vi "Process.vi"(8 "error in":errorcluster, 11 "Measurement.WavelengthSweeping.UI":refnum<class "Measurement.WavelengthSweeping.UI.lvclass">) -> (0 "error out":errorcluster, 3 "Measurement.WavelengthSweeping.UI out":refnum<class "Measurement.WavelengthSweeping.UI.lvclass">)   [LabVIEW 2017, in "Measurement.WavelengthSweeping.UI.lvclass"]
doc: "---------------------------------------------------------------\nJKI State Machine Objects™\nhttp://jki.net/state-machine-objects/\nCopyright (C) 2005-2015, JKI <info@jki.net>\nALL RIGHTS RESERVEDJKI State Machine Objects (SMO) 1.0.0.5\nJKI - JKI\nCopyright (c) 2016, JKI"
uses:
  Measurement.WavelengthSweeping.UI.lvclass
  D:/Program Files (x86)/National Instruments/LabVIEW 2017/vi.lib/JKI/JKI SMO/SMO/SMO.lvclass
  D:/Program Files (x86)/National Instruments/LabVIEW 2017/vi.lib/JKI/JKI SMO/SMO.UI/SMO.UI.lvclass
  <vilib>/JKI/JKI SMO/SMO/Typedefs/Parent Call--Enum.ctl
  Measurement.WavelengthSweeping/Typedefs/MeasuredData--Cluster.ctl
  Measurement.WavelengthSweeping/Measurement.WavelengthSweeping.lvclass
  D:/upwork/Laser Measurement Tool/Laser/project/Subsystems/Measurement/Measurement.lvclass
  Measurement.UI/Measurement.UI.lvclass
  <vilib>/JKI/JKI SMO/SMO/SMO.lvclass
  <vilib>/JKI/JKI SMO/SMO.UI/SMO.UI.lvclass
  Measurement/Measurement.lvclass
panel:
  in  "Clear Button":bool
  in  "Stop Button":bool
  in  "Pause Button":bool
  in  "Start Button":bool
  in  "Close Button":bool
  out "Initialized":bool
  out "Power monitor":cluster{"X":dbl, "Y":dbl}[](graph) caption="XY Graph - Light"
  out "SMU":cluster{"X":dbl, "Y":dbl}[](graph) caption="XY Graph - Light"
  out "LIA":cluster{"X":dbl, "Y":dbl}[](graph) caption="XY Graph - Light"
  # "For instructions on how to use the JKI State Machine Objects, examples and video tutorials, visit:\nhttp://jki.net/state-machine-objects/\n\nJKI State Machine Objects™\nhttp://jki.net/state-machine-objects/\nCopyright (C) 2005-2015, JKI <info@jki.net>\nALL RIGHTS RESERVED"
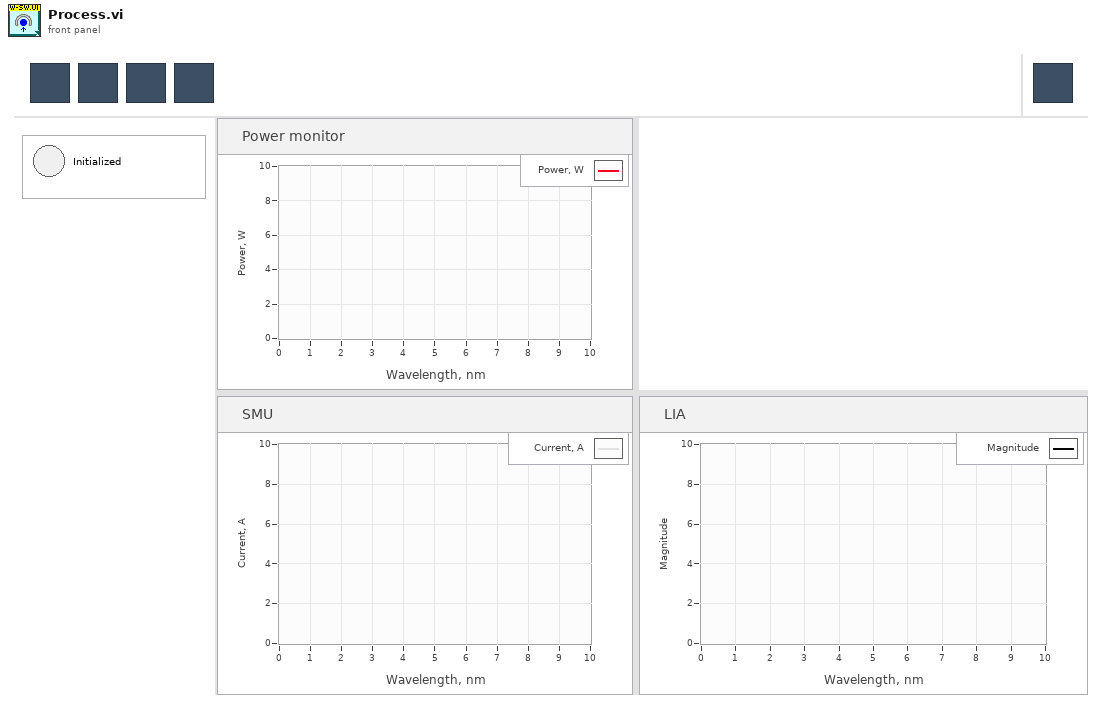
[diagram p1: front panel]
types:
  T1 = typedef "SMO.lvclass/Parent Call--Enum.ctl" = enum16{"Allows parent to run", "Does not request parent to run"}
  T2 = enum8{"Enabled", "Disabled", "Disabled and Grayed Out"}
  T3 = typedef "Measurement.WavelengthSweeping.lvclass/MeasuredData--Cluster.ctl" = cluster{"Wavelength, nm":dbl, "Power, W":dbl, "Current, A":dbl, "Magnitude":dbl}
  T4 = enum32{"invalid app kind", "Development System", "Run Time System", "Student Edition", "Embedded LabVIEW", "Evaluation", "Custom"}
  T5 = enum32{"Invalid", "Standard", "Closed", "Hidden", "Minimized", "Maximized"}
  T6 = typedef "Measurement.lvclass/PublicEvents--Measurement.Initialized.ctl" = bool
  T7 = typedef "Measurement.lvclass/PublicEvents--Measurement.Finished.ctl" = bool
  T8 = cluster{"Wavelength, nm":dbl, "Current, A":dbl}[]
  T9 = typedef "Measurement.WavelengthSweeping.UI.lvclass/Dependencies--Cluster.ctl" = cluster{"Measurement.WavelengthSweeping":refnum<class "Measurement.WavelengthSweeping.lvclass">}
  T10 = cluster{"Core":cluster{"Current VI Reference":refnum<vi>, "Close Panel on Exit?":bool, "error":errorcluster}, "Self Reference":refnum<class "Measurement.WavelengthSweeping.UI.lvclass">, "Dependencies":T9, "SMU Data":cluster{"X":dbl, "Y":dbl}[], "LIA Data":cluster{"X":dbl, "Y":dbl}[], "OPM Data":cluster{"X":dbl, "Y":dbl}[]}
  T11 = cluster{"Current VI Reference":refnum<vi>, "Close Panel on Exit?":bool, "error":errorcluster}
  T12 = typedef "SMO.lvclass/Protected Events.ctl" = cluster{"StopProcesses":refnum<user-event>, "AbortProcesses":refnum<user-event>, "Config Changed":refnum<user-event>, "Dependency":refnum<user-event>}
  T13 = cluster{"Event Registration Refnum":refnum<event-registration>, "Measurement Public Events":refnum<event-registration>}
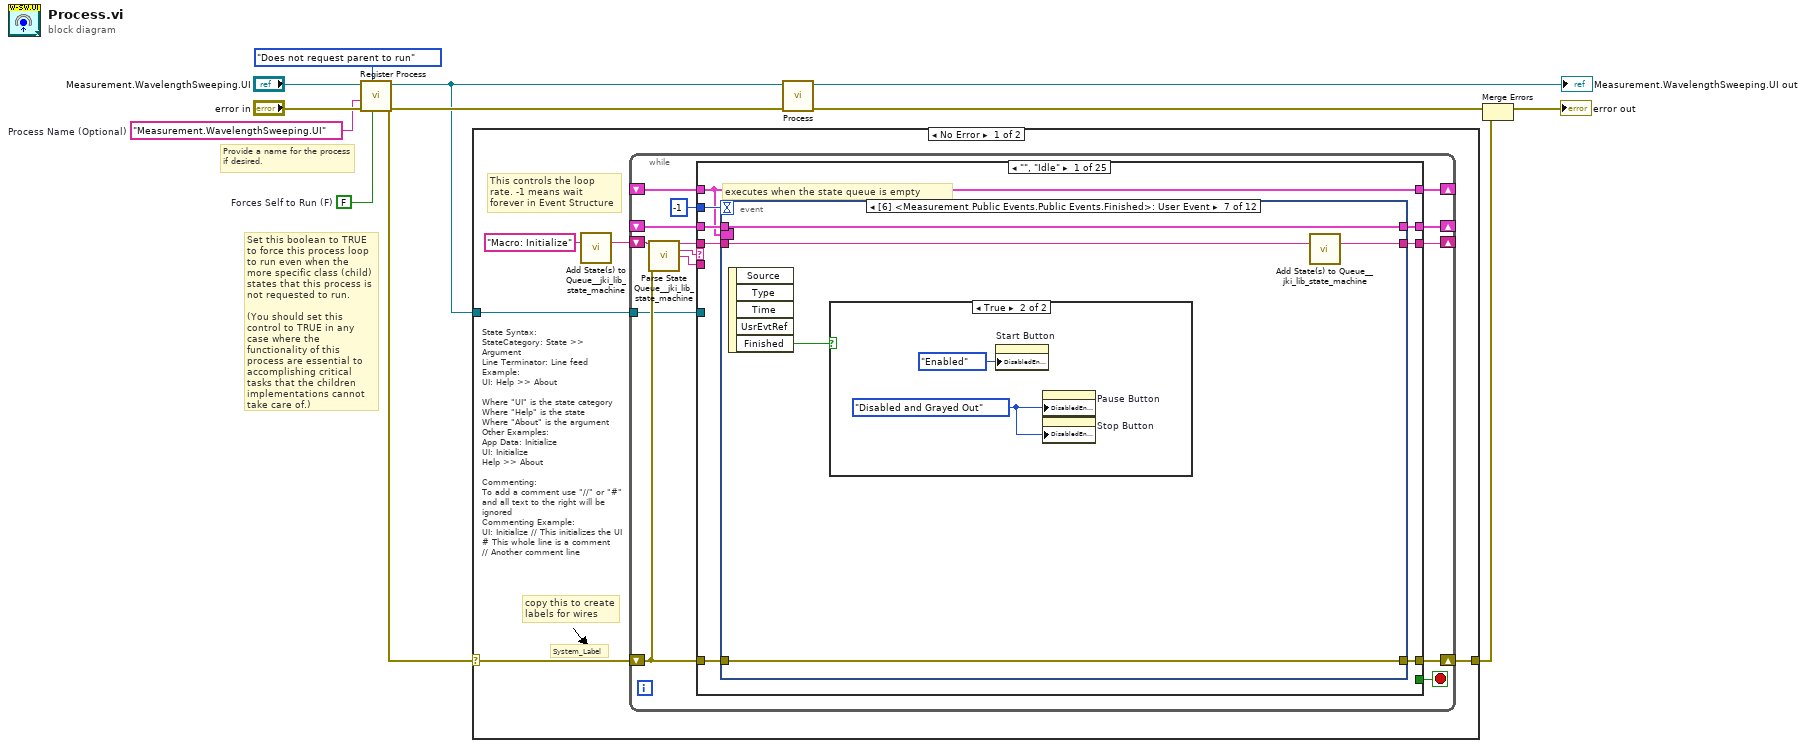
[diagram p0: block diagram]
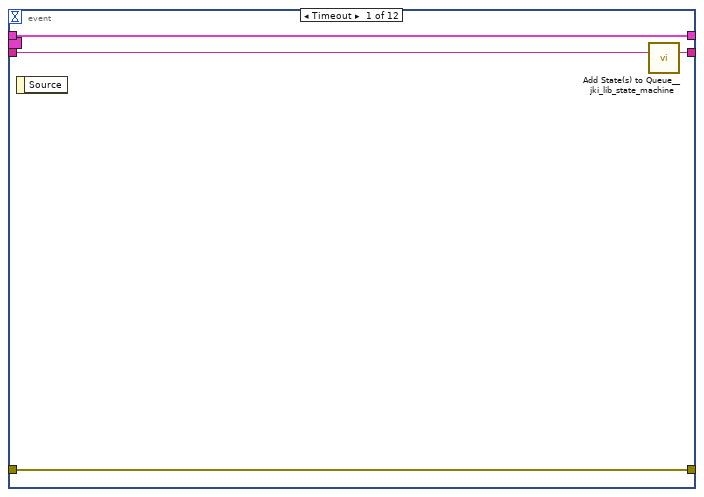
[diagram p2: hidden frame]
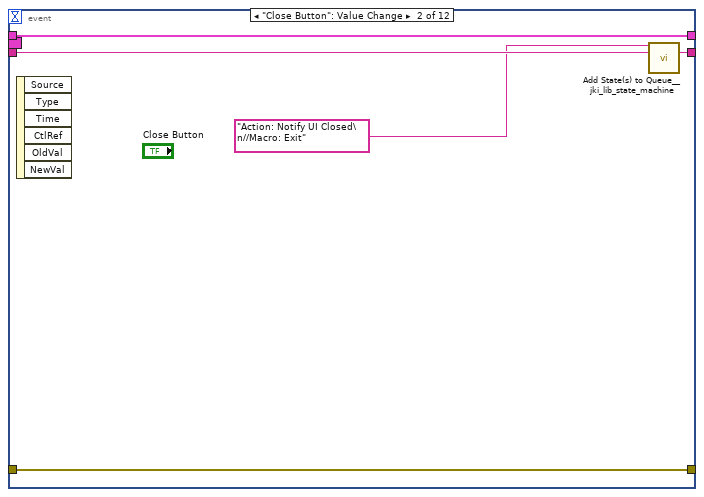
[diagram p3: hidden frame]
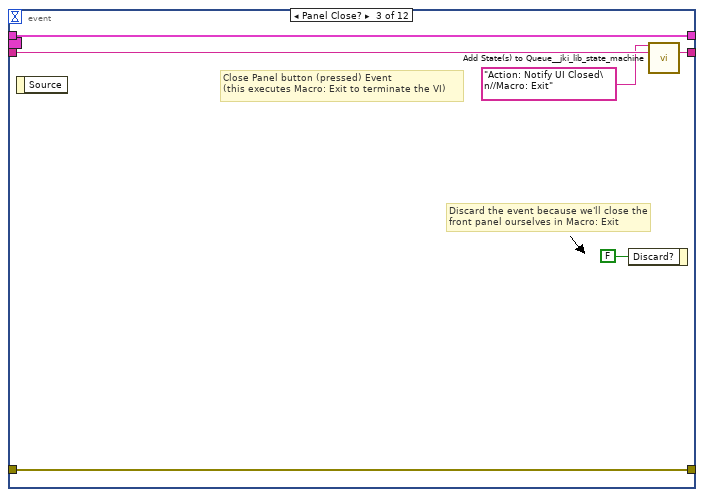
[diagram p4: hidden frame]
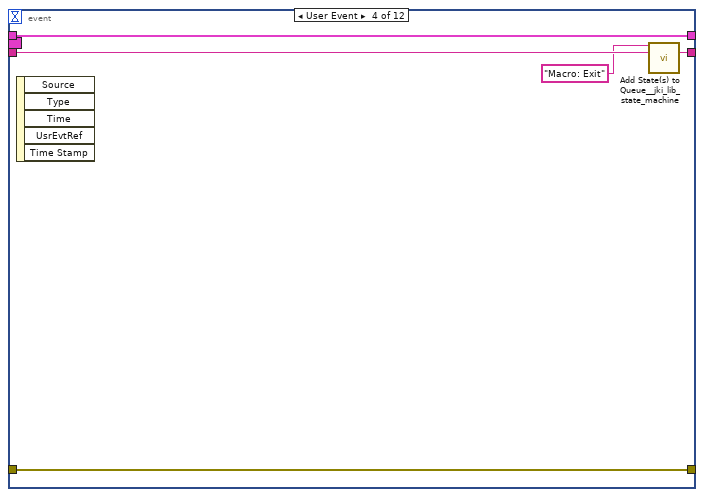
[diagram p5: hidden frame]
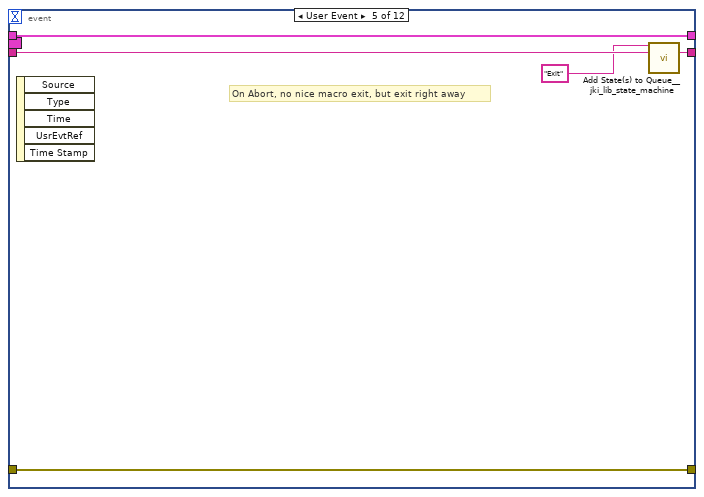
[diagram p6: hidden frame]
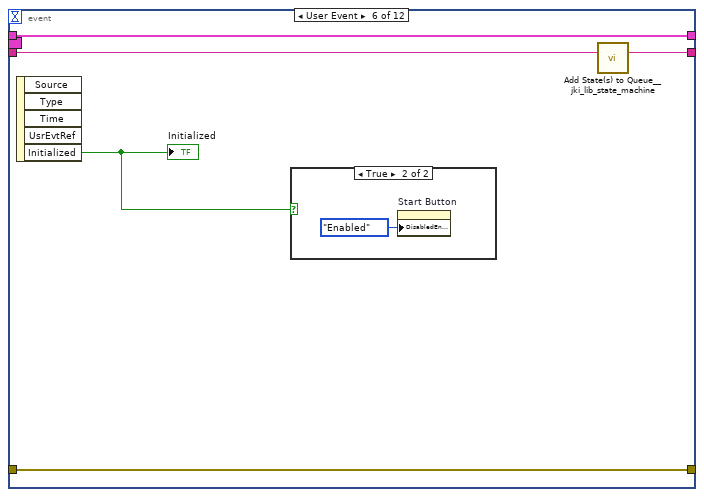
[diagram p7: hidden frame]
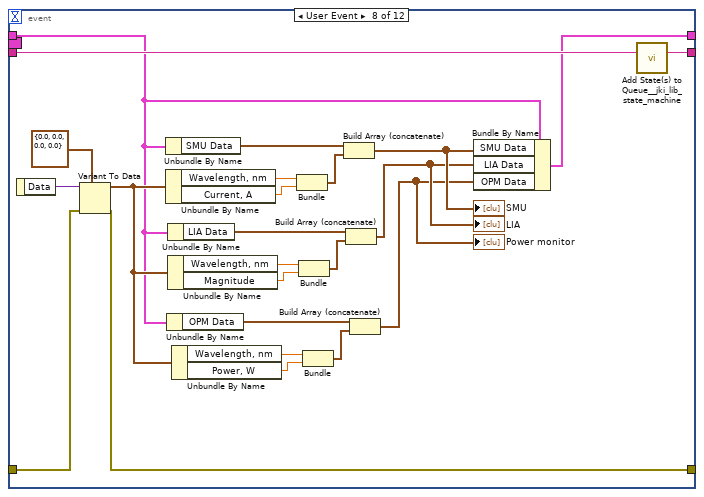
[diagram p10: hidden frame]
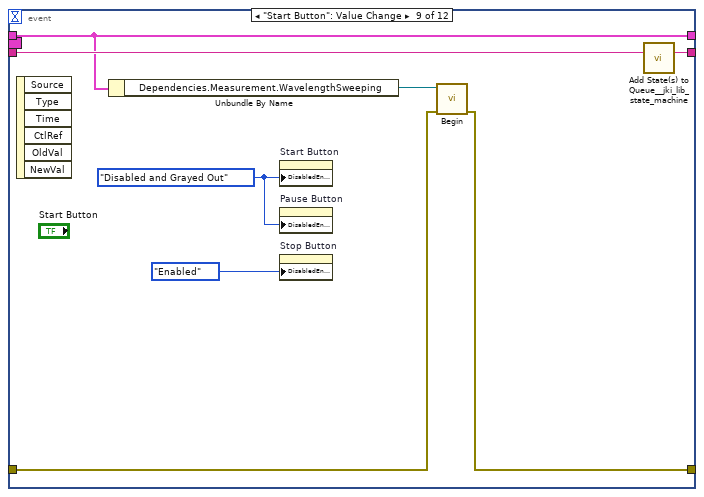
[diagram p11: hidden frame]
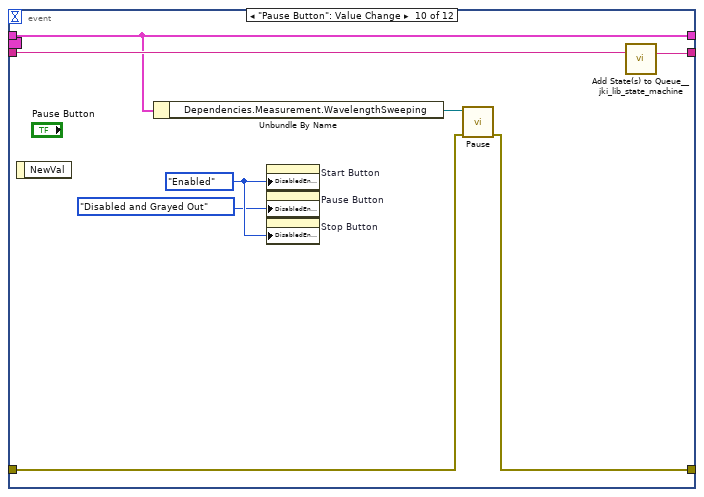
[diagram p12: hidden frame]
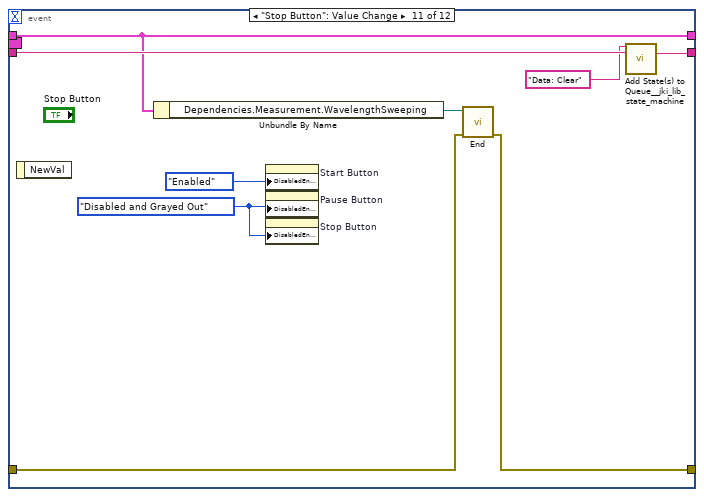
[diagram p13: hidden frame]
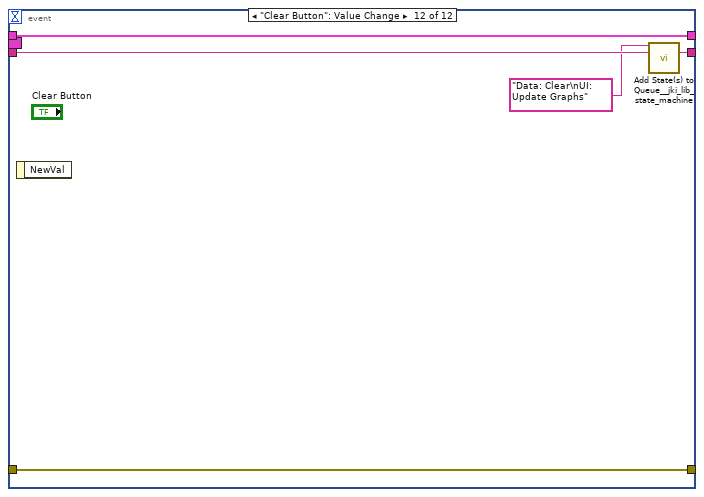
[diagram p14: hidden frame]
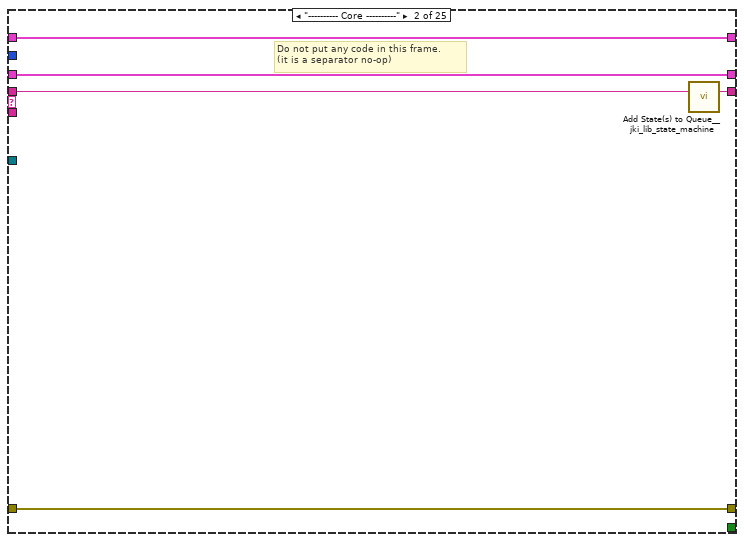
[diagram p15: hidden frame]
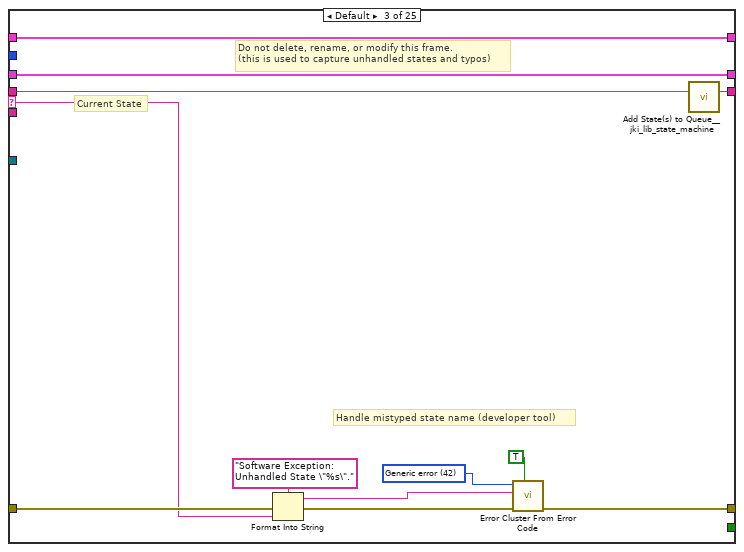
[diagram p16: hidden frame]
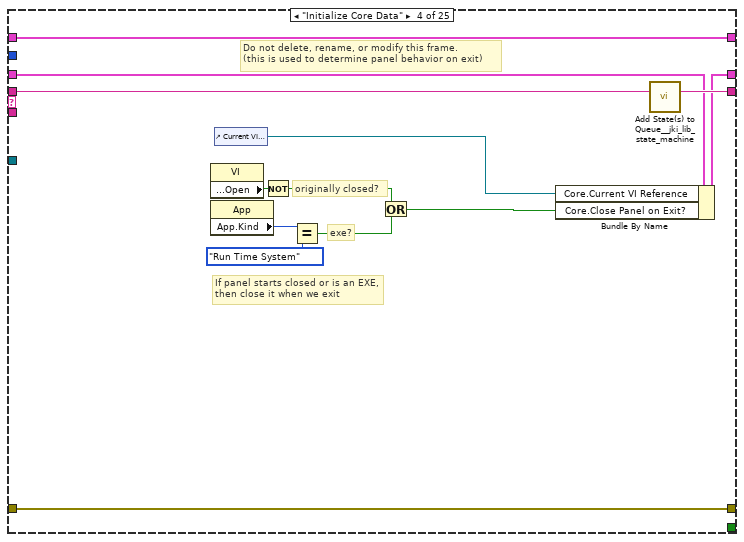
[diagram p17: hidden frame]
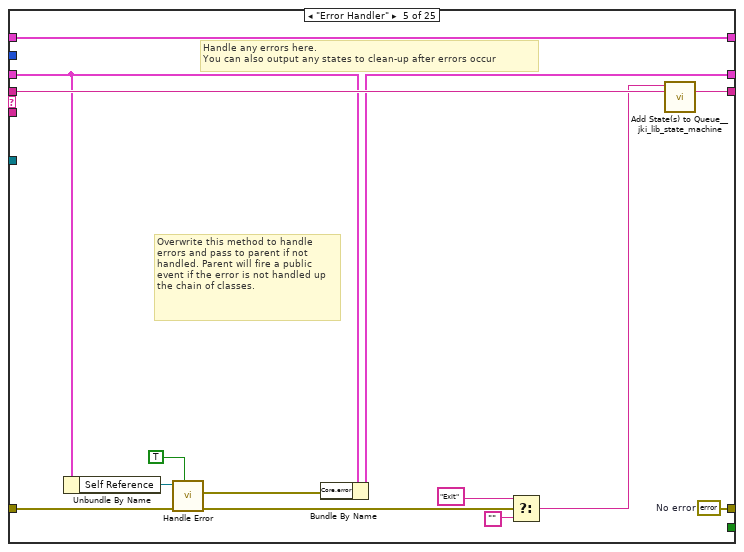
[diagram p18: hidden frame]
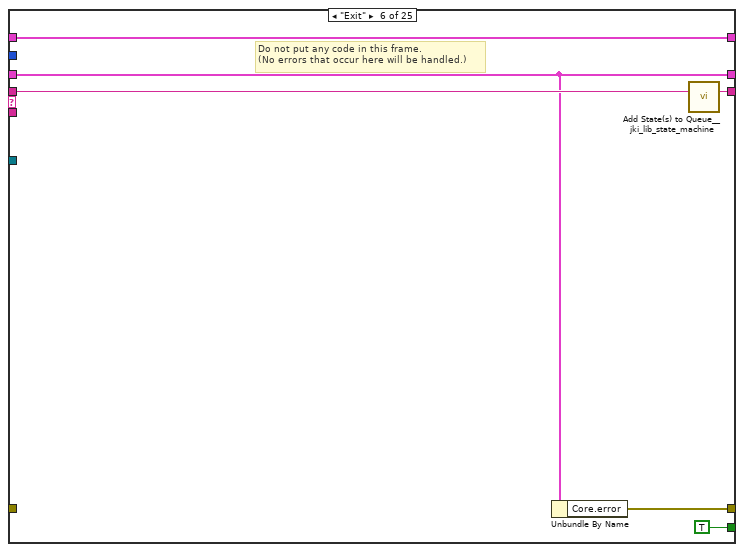
[diagram p19: hidden frame]
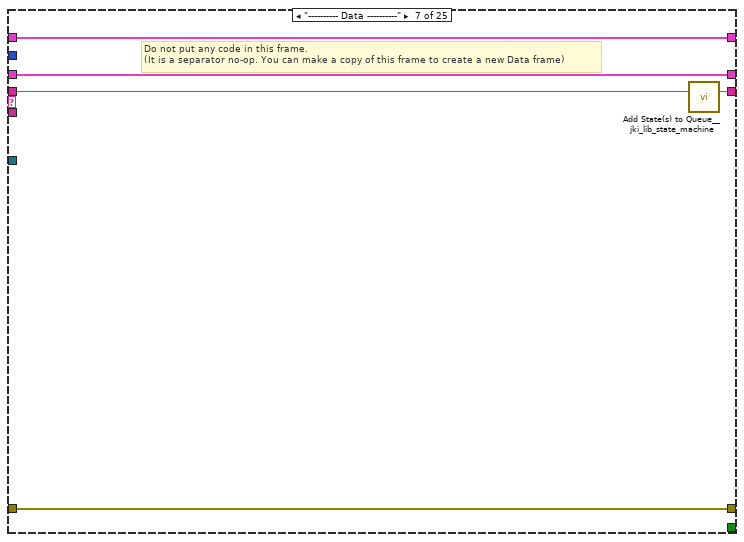
[diagram p20: hidden frame]
diagram:
  w2 = FALSE  # Forces Self to Run (F)
  w1 = "Measurement.WavelengthSweeping.UI"  # Process Name (Optional)
  # "Provide a name for the process\nif desired."
  # "Set this boolean to TRUE to force this process loop to run even when the more specific class (child) states that this process is not requested to run.\n\n(You should set this control to TRUE in any case where the functionality of this process are essential to accomplishing critical tasks that the children implementations cannot take care of.)"
  n1 = call <vilib>:"Register Process.vi"("Forces Self to Run (F)"=w2, "Parent Call"=Parent_Call--Enum."Does not request parent to run", "error in (no error)"="error in", "Process Name (optional)"=w1, "SMO"="Measurement.WavelengthSweeping.UI") -> ("error out"=w8:errorcluster, "SMO out"=w7:refnum<class "Measurement.WavelengthSweeping.UI.lvclass">)  [unwired: 5 in]
  n2 = case shown="No Error" w8 {
    selector: w8 -> [w13 w375]
    tunnel: w7 -> [w14 _]
    tunnel: [w12 w375] -> w4
    frame No Error {
      # "State Syntax:\nStateCategory: State >> Argument\nLine Terminator: Line feed\nExample:\nUI: Help >> About\n\nWhere \"UI\" is the state category\nWhere \"Help\" is the state\nWhere \"About\" is the argument\nOther Examples:\nApp Data: Initialize\nUI: Initialize\nHelp >> About\n\nCommenting:\nTo add a comment use \"//\" or \"#\" and all text to the right will be ignored\nCommenting Example:\nUI: Initialize // This initializes the UI\n# This whole line is a comment\n// Another comment line"
      # "copy this to create labels for wires"
      # "This controls the loop rate. -1 means wait forever in Event Structure"
      # "System_Label"
      n3 = call <vilib>:"Add State(s) to Queue__jki_lib_state_machine.vi"("State(s) in (\"\")"="Macro: Initialize") -> ("States Out"=w16:string)  [unwired: 14 in]
      n4 = while {
        shift-right: [w23] -> _
        shift-left: _ -> [w22]
        shift-right: [w26] -> w12
        shift-left: w13 -> [w20]
        shift-right: [w25] -> _
        shift-left: w16 -> [w27]
        tunnel: w14 -> [w19]
        shift-right: [w18] -> _
        shift-left: _ -> [w17]
        stop <- w24 stop-if-true
        n5 = call <vilib>:"Parse State Queue__jki_lib_state_machine.vi"("State Queue"=w27, "Error In (no error)"=w20) -> ("Remaining States"=w29:string, "Current State"=w30:string, "Arguments"=w28:string)  [unwired: 11 in]
        n6 = case shown="\"\", \"Idle\"" w30 {
          selector: w30 -> [_ _ w137 _ _ _ _ _ _ _ _ _ _ _ _ _ _ _ _ _ _ _ _ _ _]
          tunnel: w29 -> [w38 w135 w141 w160 w174 w180 w185 w200 w205 w214 w219 w229 w236 w252 w291 w296 w305 w319 w324 w335 w340 w354 w360 w367 w374]
          tunnel: w28 -> [_ _ _ _ _ _ _ _ _ _ _ _ w230 w246 _ _ _ _ _ _ _ _ _ _ _]
          tunnel: w22 -> [w36 w132 w139 w151 w163 w176 w182 _ w204 w209 w216 w227 w234 w248 w288 w293 w301 w310 w321 w332 w337 w346 w358 w363 w370]
          tunnel: [w35 w133 w143 w157 w165 w175 w183 w189 w202 w210 w217 w221 w231 w249 w280 w294 w303 w317 w322 w326 w338 w348 w355 w364 w368] -> w26
          tunnel: w20 -> [w34 w133 w142 w157 w170 _ w183 w197 w202 w211 w217 w225 w232 w250 w284 w294 w303 w317 w322 w327 w338 w350 w356 w364 w369]
          tunnel: [w37 w134 w140 w159 w173 w179 w184 w199 w206 w213 w218 w228 w235 w251 w290 w295 w304 w318 w323 w334 w339 w353 w359 w366 w373] -> w25
          tunnel: [_ _ _ _ _ TRUE _ _ _ _ _ _ _ _ _ _ _ _ _ _ _ _ _ _ _] -> w24
          tunnel: [w33 w132 w139 w158 w162 w176 w182 w198 w203 w209 w216 w227 w234 w248 w288 w293 w301 w310 w321 w332 w337 w346 w358 w362 w370] -> w23
          tunnel: -1 ("Timeout") -> [w32 _ _ _ _ _ _ _ _ _ _ _ _ _ _ _ _ _ _ _ _ _ _ _ _]
          tunnel: w19 -> [_ _ _ _ _ _ _ w195 _ _ _ _ _ _ _ _ _ _ _ _ _ _ _ _ _]
          tunnel: [w31 w131 w136 w148 w172 w177 w181 w194 w207 w208 w215 w226 w233 w245 w289 w292 w302 w311 w320 w333 w336 w343 w357 w365 w372] -> w18
          tunnel: w17 -> [w31 w131 w136 w148 w172 w177 w181 w194 w207 w208 w215 w226 w233 w245 w289 w292 w302 w311 w320 w333 w336 _ w357 w365 w372]
          frame "", "Idle" {
            # "executes when the state queue is empty"
            n7 = event shown="[6] <Measurement Public Events.Public Events.Finished>: User Event" {
              selector: w31 -> [_ _ _ _ _ _ _ _ _ _ _ _]
              dyn-events: _ -> [_ _ _ _ _ _ _ _ _ _ _ _]
              timeout: w32 -> [_ _ _ _ _ _ _ _ _ _ _ _]
              tunnel: w38 -> [w42 w47 w53 w58 w63 w65 w71 w99 w107 w115 w124 w130]
              tunnel: [w41 w46 w52 w57 w62 w66 w72 w100 w108 w116 w125 w129] -> w37
              tunnel: w36 -> [w39 w44 w49 w55 w60 w67 w73 w81 w106 w114 w123 w127]
              tunnel: [w40 w45 w48 w56 w61 w68 w74 w96 w103 w111 w120 w128] -> w35
              tunnel: w34 -> [w40 w45 w48 w56 w61 w68 w74 w97 w104 w112 w121 w128]
              tunnel: [w39 w44 w49 w55 w60 w67 w73 w80 w106 w114 w123 w127] -> w33
              event Timeout {
                n8 = event-data() -> ()  [unwired: 1 in, 1 out]
                n9 = call <vilib>:"Add State(s) to Queue__jki_lib_state_machine.vi"("State(s) in (\"\")"=w42) -> ("States Out"=w41:string)  [unwired: 14 in]
              }
              event "Close Button": Value Change {
                n10 = event-data() -> ()  [unwired: 1 in, 6 out]
                n11 = call <vilib>:"Add State(s) to Queue__jki_lib_state_machine.vi"("State(s) in Front (\"\")"="Action: Notify UI Closed\n//Macro: Exit" ("State(s) in Front (\"\")"), "State(s) in (\"\")"=w47) -> ("States Out"=w46:string)  [unwired: 13 in]
              }
              event Panel Close? {
                # "Discard the event because we'll close the front panel ourselves in Macro: Exit"
                # "Close Panel button (pressed) Event\n(this executes Macro: Exit to terminate the VI)"
                n12 = event-data() -> ()  [unwired: 1 in, 1 out]
                n13 = event-data("Discard?"=FALSE) -> ()  [unwired: 1 in, 1 out]
                n14 = call <vilib>:"Add State(s) to Queue__jki_lib_state_machine.vi"("State(s) in Front (\"\")"="Action: Notify UI Closed\n//Macro: Exit", "State(s) in (\"\")"=w53) -> ("States Out"=w52:string)  [unwired: 13 in]
              }
              event User Event {
                n15 = event-data() -> ()  [unwired: 1 in, 5 out]
                n16 = call <vilib>:"Add State(s) to Queue__jki_lib_state_machine.vi"("State(s) in Front (\"\")"="Macro: Exit", "State(s) in (\"\")"=w58) -> ("States Out"=w57:string)  [unwired: 13 in]
              }
              event User Event {
                # "On Abort, no nice macro exit, but exit right away"
                n17 = event-data() -> ()  [unwired: 1 in, 5 out]
                n18 = call <vilib>:"Add State(s) to Queue__jki_lib_state_machine.vi"("State(s) in Front (\"\")"="Exit", "State(s) in (\"\")"=w63) -> ("States Out"=w62:string)  [unwired: 13 in]
              }
              event User Event {
                n19 = event-data() -> ("Initialized"=w64:T6)  [unwired: 1 in, 4 out]
                "Initialized" <- w64
                n20 = case shown="True" w64 {
                  frame False {
                  }
                  frame True {
                    n21 = property on="Start Button" class="Bool"("DisabledEnum"=T2."Enabled" ("Disabled")) -> ()  [unwired: 2 in, 2 out]
                  }
                }
                n22 = call <vilib>:"Add State(s) to Queue__jki_lib_state_machine.vi"("State(s) in (\"\")"=w65) -> ("States Out"=w66:string)  [unwired: 14 in]
              }
              event User Event {
                n23 = event-data() -> ("Finished"=w70:T7)  [unwired: 1 in, 4 out]
                n24 = case shown="True" w70 {
                  frame False {
                  }
                  frame True {
                    w75 = T2."Disabled and Grayed Out" ("Disabled")
                    n25 = property on="Start Button" class="Bool"("DisabledEnum"=T2."Enabled" ("Disabled")) -> ()  [unwired: 2 in, 2 out]
                    n26 = property on="Pause Button" class="Bool"("DisabledEnum"=w75) -> ()  [unwired: 2 in, 2 out]
                    n27 = property on="Stop Button" class="Bool"("DisabledEnum"=w75) -> ()  [unwired: 2 in, 2 out]
                  }
                }
                n28 = call <vilib>:"Add State(s) to Queue__jki_lib_state_machine.vi"("State(s) in (\"\")"=w71) -> ("States Out"=w72:string)  [unwired: 14 in]
              }
              event User Event {
                n29 = event-data() -> ("Data"=w98:variant)  [unwired: 1 in]
                n30 = Variant To Data(error in=w97, type=T3 {"Wavelength, nm"=0.0, "Power, W"=0.0, "Current, A"=0.0, "Magnitude"=0.0} ("Measured Data"), Variant=w98) -> (data=w82:T3, error out=w96:errorcluster)
                n31 = Unbundle By Name(w81) -> ("SMU Data"=w92:cluster{"X":dbl, "Y":dbl}[])
                n32 = Unbundle By Name(w82) -> ("Wavelength, nm"=w94:dbl, "Current, A"=w93:dbl)
                n33 = Unbundle By Name(w81) -> ("OPM Data"=w84:cluster{"X":dbl, "Y":dbl}[])
                n34 = Unbundle By Name(w81) -> ("LIA Data"=w89:cluster{"X":dbl, "Y":dbl}[])
                n35 = Unbundle By Name(w82) -> ("Wavelength, nm"=w87:dbl, "Magnitude"=w88:dbl)
                n36 = Unbundle By Name(w82) -> ("Wavelength, nm"=w86:dbl, "Power, W"=w85:dbl)
                n37 = Bundle("Wavelength, nm"=w94, "Current, A"=w93) -> (w91:cluster{"Wavelength, nm":dbl, "Current, A":dbl})  [unwired: 1 in]
                n38 = Bundle("Wavelength, nm"=w87, "Magnitude"=w88) -> (w90:cluster{"Wavelength, nm":dbl, "Magnitude":dbl})  [unwired: 1 in]
                n39 = Bundle("Wavelength, nm"=w86, "Power, W"=w85) -> (w83:cluster{"Wavelength, nm":dbl, "Power, W":dbl})  [unwired: 1 in]
                n40 = Build Array (concatenate)(w92, w91) -> (w79:T8)
                "SMU" <- w79
                n41 = Build Array (concatenate)(w89, w90) -> (w78:cluster{"Wavelength, nm":dbl, "Magnitude":dbl}[])
                "LIA" <- w78
                n42 = Build Array (concatenate)(w84, w83) -> (w77:cluster{"Wavelength, nm":dbl, "Power, W":dbl}[])
                "Power monitor" <- w77
                n43 = Bundle By Name(cluster=w81, "SMU Data"=w79, "LIA Data"=w78, "OPM Data"=w77) -> (w80:T10)
                n44 = call <vilib>:"Add State(s) to Queue__jki_lib_state_machine.vi"("State(s) in (\"\")"=w99) -> ("States Out"=w100:string)  [unwired: 14 in]
              }
              event "Start Button": Value Change {
                w101 = T2."Disabled and Grayed Out" ("Disabled")
                n45 = event-data() -> ()  [unwired: 1 in, 6 out]
                n46 = Unbundle By Name(w106) -> ("Dependencies.Measurement.WavelengthSweeping"=w105:refnum<class "Measurement.WavelengthSweeping.lvclass">)
                n47 = property on="Start Button" class="Bool"("DisabledEnum"=w101) -> ()  [unwired: 2 in, 2 out]
                n48 = property on="Pause Button" class="Bool"("DisabledEnum"=w101) -> ()  [unwired: 2 in, 2 out]
                n49 = property on="Stop Button" class="Bool"("DisabledEnum"=T2."Enabled" ("Disabled")) -> ()  [unwired: 2 in, 2 out]
                n50 = call "Begin.vi"("error in (no error)"=w104, "Measurement in"=w105) -> ("error out"=w103:errorcluster)  [unwired: 8 in, 1 out]
                n51 = call <vilib>:"Add State(s) to Queue__jki_lib_state_machine.vi"("State(s) in (\"\")"=w107) -> ("States Out"=w108:string)  [unwired: 14 in]
              }
              event "Pause Button": Value Change {
                w110 = T2."Enabled" ("Disabled")
                n52 = event-data() -> ()  [unwired: 1 in, 1 out]
                n53 = Unbundle By Name(w114) -> ("Dependencies.Measurement.WavelengthSweeping"=w113:refnum<class "Measurement.WavelengthSweeping.lvclass">)
                n54 = property on="Start Button" class="Bool"("DisabledEnum"=w110) -> ()  [unwired: 2 in, 2 out]
                n55 = property on="Pause Button" class="Bool"("DisabledEnum"=T2."Disabled and Grayed Out" ("Disabled")) -> ()  [unwired: 2 in, 2 out]
                n56 = property on="Stop Button" class="Bool"("DisabledEnum"=w110) -> ()  [unwired: 2 in, 2 out]
                n57 = call "Pause.vi"("error in (no error)"=w112, "Measurement in"=w113) -> ("error out"=w111:errorcluster)  [unwired: 8 in, 1 out]
                n58 = call <vilib>:"Add State(s) to Queue__jki_lib_state_machine.vi"("State(s) in (\"\")"=w115) -> ("States Out"=w116:string)  [unwired: 14 in]
              }
              event "Stop Button": Value Change {
                w118 = T2."Disabled and Grayed Out" ("Disabled")
                n59 = event-data() -> ()  [unwired: 1 in, 1 out]
                n60 = Unbundle By Name(w123) -> ("Dependencies.Measurement.WavelengthSweeping"=w122:refnum<class "Measurement.WavelengthSweeping.lvclass">)
                n61 = property on="Start Button" class="Bool"("DisabledEnum"=T2."Enabled" ("Disabled")) -> ()  [unwired: 2 in, 2 out]
                n62 = property on="Pause Button" class="Bool"("DisabledEnum"=w118) -> ()  [unwired: 2 in, 2 out]
                n63 = property on="Stop Button" class="Bool"("DisabledEnum"=w118) -> ()  [unwired: 2 in, 2 out]
                n64 = call "End.vi"("error in (no error)"=w121, "Measurement in"=w122) -> ("error out"=w120:errorcluster)  [unwired: 8 in, 1 out]
                n65 = call <vilib>:"Add State(s) to Queue__jki_lib_state_machine.vi"("State(s) in Front (\"\")"="Data: Clear", "State(s) in (\"\")"=w124) -> ("States Out"=w125:string)  [unwired: 13 in]
              }
              event "Clear Button": Value Change {
                n66 = event-data() -> ()  [unwired: 1 in, 1 out]
                n67 = call <vilib>:"Add State(s) to Queue__jki_lib_state_machine.vi"("State(s) in Front (\"\")"="Data: Clear\nUI: Update Graphs", "State(s) in (\"\")"=w130) -> ("States Out"=w129:string)  [unwired: 13 in]
              }
            }
          }
          frame "---------- Core ----------" {
            # "Do not put any code in this frame.\n(it is a separator no-op)"
            n68 = call <vilib>:"Add State(s) to Queue__jki_lib_state_machine.vi"("State(s) in (\"\")"=w135) -> ("States Out"=w134:string)  [unwired: 14 in]
          }
          frame Default {
            w146 = 42 items=["No error", "Argument error", "Memory is full", "Out of zone", "End of file", "File already open", "Generic file I/O error", "File not found", "File permission error", "Disk is full", "Duplicate path", "Too many files open", "System feature not enabled", "Resource file not found", "Cannot add resource", "Resource not found", "Image not found", "Image memory error", "Pen does not exist", "Config type invalid", "Config token not found", "Config parse error", "Config memory error", "Bad external code format", "Bad external code offset", "External code not present", "Null window", "Destroy window error", "Null menu", "Print aborted", "Bad print record", "Print driver error", "Windows error during printing", "Memory error during printing", "Print dialog error", "Generic print error", "Invalid device refnum", "Device not found", "Device parameter error", "Device unit error", "Cannot open device", "Device call aborted", "Generic error", "Cancelled by user", "Object ID too low", "Object ID too high", "Object not in heap", "Unknown heap", "Unknown object (invalid DefProc)", "Unknown object (DefProc not in table)", "Message out of range", "Invalid (null) method", "Unknown message", "Manager call not supported", "Bad address", "Network operation in progress", "Network operation timed out", "Connection is busy", "Network attribute not supported", "Network error", "Address in use", "System out of memory", "Connection aborted", "Connection refused", "Not connected", "Already connected", "Connection closed", "Initialization error (interapplication manager)", "Bad occurrence", "Wait on unbound occurrence handler", "Occurrence queue overflow", "Datalog type conflict", "Unused", "Unrecognized type (interapplication manager)", "Memory corrupt", "Failed to make temporary DLL", "Old CIN version", "Drag socket not found", "Failed to load drop-object", "Failed to register OLE object", "Failed to release OLE object", "Format specifier type mismatch", "Unknown format specifier", "Too few format specifiers", "Too many format specifiers", "Scan failed", "Newer CIN version", "Error converting to variant", "Runtime menu error", "Password tampered", "Variant attribute not found", "Incompatible variant data type", "Event data is not available", "Event Store is not present", "Occurrence is not found", "Event Queue is not created", "Event info is not available", "Refnum passed is NULL", "Error retrieving Class GUID", "Error retrieving CoClass GUID", "Error retrieving TypeLib GUID.", "Bad built application magic bytes.", "Specific driver is different from the specific driver associated with the Logical Name.", "There is no session opened to the class driver.", "Max Error", "MAX - Error with config objects", "MAX - Error loading configuration", "MAX - Group not supported"]
            # "Current State"
            # "Do not delete, rename, or modify this frame.\n(this is used to capture unhandled states and typos)"
            # "Handle mistyped state name (developer tool)"
            n69 = Format Into String(format string="Software Exception: Unhandled State \"%s\"." ("message"), error in=w142, w137) -> (resulting string=w145:string, error out=w144:errorcluster)  [unwired: 1 in]
            n70 = call <vilib>:"Error Cluster From Error Code.vi"("show call chain? (False)"=TRUE, "error in (no error)"=w144, "error message (\"\")"=w145, "error code (0)"=w146) -> ("error out"=w143:errorcluster)  [unwired: 5 in]
            n71 = call <vilib>:"Add State(s) to Queue__jki_lib_state_machine.vi"("State(s) in (\"\")"=w141) -> ("States Out"=w140:string)  [unwired: 14 in]
          }
          frame "Initialize Core Data" {
            # "Do not delete, rename, or modify this frame.\n(this is used to determine panel behavior on exit)"
            # "originally closed?"
            # "exe?"
            # "If panel starts closed or is an EXE, then close it when we exit"
            n72 = property class="VI"() -> ("Front Panel.Open"=w156:bool)  [unwired: 2 in, 2 out]
            n73 = property class="App"() -> ("App.Kind"=w155:T4)  [unwired: 2 in, 2 out]
            n74 = control-ref of="Current VI Reference"() -> (w149:refnum<vi>)
            n75 = Not(x=w156) -> (.not. x?=w153:bool)
            n76 = Equal?(x=w155, y=T4."Run Time System" ("Application:Kind")) -> (x = y?=w152:bool)
            n77 = Or(x=w153, y=w152) -> (x .or. y?=w150:bool)
            n78 = Bundle By Name(cluster=w151, "Core.Current VI Reference"=w149, "Core.Close Panel on Exit?"=w150) -> (w158:T10)
            n79 = call <vilib>:"Add State(s) to Queue__jki_lib_state_machine.vi"("State(s) in (\"\")"=w160) -> ("States Out"=w159:string)  [unwired: 14 in]
          }
          frame "Error Handler" {
            w165 = errorcluster {"status"=FALSE, "code"=0, "source"=""}  # No error
            # "Overwrite this method to handle errors and pass to parent if not handled. Parent will fire a public event if the error is not handled up the chain of classes."
            # "Handle any errors here.\nYou can also output any states to clean-up after errors occur"
            n80 = Unbundle By Name(w163) -> ("Self Reference"=w171:refnum<class "Measurement.WavelengthSweeping.UI.lvclass">)
            n81 = call-dynamic "Handle Error.vi"("Stop on Unhandled Error (T)"=TRUE, "error in"=w170, "SMO"=w171) -> ("handling error"=w166:errorcluster, "Unhandled error"=w164:errorcluster)  [unwired: 6 in, 1 out]
            n82 = Bundle By Name(cluster=w163, "Core.error"=w164) -> (w162:T10)
            n83 = Select(t="Exit", s=w166, f="") -> (s? t:f=w167:string)
            n84 = call <vilib>:"Add State(s) to Queue__jki_lib_state_machine.vi"("State(s) in Front (\"\")"=w167, "State(s) in (\"\")"=w174) -> ("States Out"=w173:string)  [unwired: 13 in]
          }
          frame "Exit" {
            # "Do not put any code in this frame.\n(No errors that occur here will be handled.)"
            n85 = Unbundle By Name(w176) -> ("Core.error"=w175:errorcluster)
            n86 = call <vilib>:"Add State(s) to Queue__jki_lib_state_machine.vi"("State(s) in (\"\")"=w180) -> ("States Out"=w179:string)  [unwired: 14 in]
          }
          frame "---------- Data ----------" {
            # "Do not put any code in this frame.\n(It is a separator no-op. You can make a copy of this frame to create a new Data frame)"
            n87 = call <vilib>:"Add State(s) to Queue__jki_lib_state_machine.vi"("State(s) in (\"\")"=w185) -> ("States Out"=w184:string)  [unwired: 14 in]
          }
          frame "Data: Initialize" {
            w186 = cluster{"X":dbl, "Y":dbl}[] []  # OPM Data
            w187 = cluster{"X":dbl, "Y":dbl}[] []  # LIA Data
            w188 = cluster{"X":dbl, "Y":dbl}[] []  # SMU Data
            w193 = T11 {"Current VI Reference"=refnum, "Close Panel on Exit?"=FALSE, "error"={"status"=FALSE, "code"=0, "source"=""}}  # Core
            w196 = refnum<class "Measurement.WavelengthSweeping.UI.lvclass"> refnum  # Self Reference
            # "do not delete - used by framework"
            # "Data names and types of shift register data are defined by this bundle."
            # "Initialize the shift-register data, here.\n(data names are defined by what you wire into the bundle function)"
            n88 = Variant To Data(error in=w197, type=w196, Variant=w195) -> (data=w192:refnum<class "Measurement.WavelengthSweeping.UI.lvclass">, error out=w190:errorcluster)
            n89 = call "Measurement.WavelengthSweeping.UI.GetDependencies.vi"("error in (no error)"=w190, "Measurement.WavelengthSweeping.UI in"=w192) -> ("error out"=w189:errorcluster, "Dependencies"=w191:T9)  [unwired: 7 in, 1 out]
            n90 = Bundle("Core"=w193, "Self Reference"=w192, "Dependencies"=w191, "SMU Data"=w188, "LIA Data"=w187, "OPM Data"=w186) -> (w198:T10)  [unwired: 1 in]
            n91 = call <vilib>:"Add State(s) to Queue__jki_lib_state_machine.vi"("State(s) in (\"\")"=w200) -> ("States Out"=w199:string)  [unwired: 14 in]
          }
          frame "Data: Clear" {
            w201 = cluster{"X":dbl, "Y":dbl}[] [] ("SMU Data")
            n92 = Bundle By Name(cluster=w204, "SMU Data"=w201, "LIA Data"=w201, "OPM Data"=w201) -> (w203:T10)
            n93 = call <vilib>:"Add State(s) to Queue__jki_lib_state_machine.vi"("State(s) in (\"\")"=w205) -> ("States Out"=w206:string)  [unwired: 14 in]
          }
          frame "Data: Cleanup" {
            # "Cleanup any data and references, here.\n(this is called automatically, by the Macro: Exit)"
            n94 = Unbundle By Name(w209) -> ("Core.Current VI Reference"=w212:refnum<vi>)
            n95 = Close Reference(reference=w212, error in (no error)=w211) -> (error out=w210:errorcluster)
            n96 = call <vilib>:"Add State(s) to Queue__jki_lib_state_machine.vi"("State(s) in (\"\")"=w214) -> ("States Out"=w213:string)  [unwired: 14 in]
          }
          frame "---------- UI ----------" {
            # "Do not put any code in this frame.\n(It is a separator no-op. You can make a copy of this frame to create a new UI frame)"
            n97 = call <vilib>:"Add State(s) to Queue__jki_lib_state_machine.vi"("State(s) in (\"\")"=w219) -> ("States Out"=w218:string)  [unwired: 14 in]
          }
          frame "UI: Initialize" {
            w220 = T2."Disabled and Grayed Out" ("Disabled")
            # "Initialize the User Interface, here.\n(this is called automatically, by the Macro: Init)"
            n98 = invoke on="Initialized" class="Bool (strict)" method="Reinit To Default"(error in=w225) -> (error out=w222:errorcluster)  [unwired: 2 in, 2 out]
            n99 = invoke on="Power monitor" class="XYGraph (strict)" method="Reinit To Default"(error in=w222) -> (error out=w224:errorcluster)  [unwired: 2 in, 2 out]
            n100 = property on="Start Button" class="Bool"("DisabledEnum"=w220) -> ()  [unwired: 2 in, 2 out]
            n101 = property on="Pause Button" class="Bool"("DisabledEnum"=w220) -> ()  [unwired: 2 in, 2 out]
            n102 = property on="Stop Button" class="Bool"("DisabledEnum"=w220) -> ()  [unwired: 2 in, 2 out]
            n103 = invoke on="SMU" class="XYGraph (strict)" method="Reinit To Default"(error in=w224) -> (error out=w223:errorcluster)  [unwired: 2 in, 2 out]
            n104 = invoke on="LIA" class="XYGraph (strict)" method="Reinit To Default"(error in=w223) -> (error out=w221:errorcluster)  [unwired: 2 in, 2 out]
            n105 = call <vilib>:"Add State(s) to Queue__jki_lib_state_machine.vi"("State(s) in (\"\")"=w229) -> ("States Out"=w228:string)  [unwired: 14 in]
          }
          frame "UI: Cursor Set" {
            # "Argument"
            # "Initialize the User Interface, here.\n(this is called automatically, by the Macro: Init)"
            n106 = disable-structure shown="Default" {
              disable-tunnel: w232 -> [w237 w240]
              disable-tunnel: [w237 w239] -> w231
              disable-tunnel: w230 -> [_ w238]
              frame condition #0 {
              }
              frame condition #1 (active) {
                n107 = case shown="\"Idle\", Default" w238 {
                  tunnel: w240 -> [w242 w244]
                  tunnel: [w241 w243] -> w239
                  frame "Idle", Default {
                    n108 = call <vilib>:"Unset Busy.vi"("error in (no error)"=w242) -> ("error out"=w241:errorcluster)  [unwired: 10 in]
                  }
                  frame "Busy" {
                    n109 = call <vilib>:"Set Busy.vi"("error in (no error)"=w244) -> ("error out"=w243:errorcluster)  [unwired: 9 in, 1 out]
                  }
                }
              }
            }
            n110 = call <vilib>:"Add State(s) to Queue__jki_lib_state_machine.vi"("State(s) in (\"\")"=w236) -> ("States Out"=w235:string)  [unwired: 14 in]
          }
          frame "UI: Front Panel State" {
            # "Argument"
            # "Set Front Panel Open or Closed\n(Usage: \"UI: Front Panel State >> Open|Close\")"
            n111 = Unbundle By Name(w248) -> ("Core.Current VI Reference"=w247:refnum<vi>)
            n112 = disable-structure shown="Default" {
              disable-tunnel: w250 -> [w256 w279]
              disable-tunnel: [w255 w279] -> w249
              disable-tunnel: w247 -> [w254 _]
              disable-tunnel: w246 -> [w253 _]
              frame condition #0 (active) {
                n113 = case shown="\"Close\"" w253 {
                  tunnel: w256 -> [w260 w273]
                  tunnel: [w262 w274] -> w255
                  tunnel: w254 -> [w261 w271]
                  frame "Open", Default {
                    n114 = property class="VI"(reference=w261, error in=w260) -> (reference out=w258:refnum<vi>, error out=w259:errorcluster, "FP.State"=w257:T5)
                    n115 = case shown="\"Closed\"" w257 {
                      tunnel: [w265 w268] -> w262
                      tunnel: w259 -> [w264 w268]
                      tunnel: w258 -> [w263 _]
                      frame "Closed" {
                        n116 = invoke class="VI" method="FP.Open"(reference=w263, error in=w264, "Activate"=TRUE, "State"=T5."Standard") -> (error out=w265:errorcluster)  [unwired: 1 in, 4 out]
                      }
                      frame Default {
                      }
                    }
                  }
                  frame "Close" {
                    n117 = property class="VI"(reference=w271, error in=w273) -> (reference out=w270:refnum<vi>, error out=w272:errorcluster, "FP.State"=w269:T5)
                    n118 = case shown="Default" w269 {
                      tunnel: [w275 w278] -> w274
                      tunnel: w272 -> [w275 w277]
                      tunnel: w270 -> [_ w276]
                      frame "Invalid", "Closed" {
                      }
                      frame Default {
                        n119 = invoke class="VI" method="FP.Close"(reference=w276, error in=w277) -> (error out=w278:errorcluster)  [unwired: 1 in, 2 out]
                      }
                    }
                  }
                }
              }
              frame condition #1 {
              }
            }
            n120 = call <vilib>:"Add State(s) to Queue__jki_lib_state_machine.vi"("State(s) in (\"\")"=w252) -> ("States Out"=w251:string)  [unwired: 14 in]
          }
          frame "UI: Update Graphs" {
            n121 = Unbundle By Name(w288) -> ("SMU Data"=w286:cluster{"X":dbl, "Y":dbl}[], "LIA Data"=w287:cluster{"X":dbl, "Y":dbl}[], "OPM Data"=w285:cluster{"X":dbl, "Y":dbl}[])
            n122 = property on="SMU" class="XYGraph (strict)"(error in=w284, "Value"=w286) -> (error out=w283:errorcluster)  [unwired: 1 in, 1 out]
            n123 = property on="LIA" class="XYGraph (strict)"(error in=w284, "Value"=w287) -> (error out=w282:errorcluster)  [unwired: 1 in, 1 out]
            n124 = property on="Power monitor" class="XYGraph (strict)"(error in=w284, "Value"=w285) -> (error out=w281:errorcluster)  [unwired: 1 in, 1 out]
            n125 = Merge Errors(w283, w282, w281) -> (w280:errorcluster)
            n126 = call <vilib>:"Add State(s) to Queue__jki_lib_state_machine.vi"("State(s) in (\"\")"=w291) -> ("States Out"=w290:string)  [unwired: 14 in]
          }
          frame "---------- Macro ----------" {
            # "Do not put any code in this frame.\n(It is a separator no-op. You can make a copy of this frame to create a new Macro frame)"
            n127 = call <vilib>:"Add State(s) to Queue__jki_lib_state_machine.vi"("State(s) in (\"\")"=w296) -> ("States Out"=w295:string)  [unwired: 14 in]
          }
          frame "Macro: Initialize" {
            w299 = "UI: Initialize\n//UI: Front Panel State >> Open"  # UI: Initialize //UI: Front Panel State >> Open
            # "Initialization Macro\n(This is called once, when the VI starts)"
            n128 = call <vilib>:"Add State(s) to Queue__jki_lib_state_machine.vi"("State(s) in Front (\"\")"="Data: Initialize\nInitialize Core Data\nEvents: Register", "State(s) in (\"\")"="Process: Sync", "State(s) at Back (\"\")"=w299) -> ("States Out"=w298:string)  [unwired: 12 in]
            n129 = call <vilib>:"Add State(s) to Queue__jki_lib_state_machine.vi"("State(s) in Front (\"\")"=w298, "State(s) in (\"\")"=w305) -> ("States Out"=w304:string)  [unwired: 13 in]
          }
          frame "Macro: Exit" {
            # "Exit Macro\n(This is called once, when the VI exits)"
            n130 = Unbundle By Name(w310) -> ("Core.Close Panel on Exit?"=w316:bool)
            n131 = Select(t="//UI: Front Panel State >> Close", s=w316, f="") -> (s? t:f=w313:string)
            n132 = call <vilib>:"Add State(s) to Queue__jki_lib_state_machine.vi"("State(s) in Front (\"\")"="Data: Cleanup\nEvents: Unregister", "State(s) in (\"\")"="Process: Sync", "State(s) at Back (\"\")"="Exit") -> ("States Out"=w307:string)  [unwired: 12 in]
            n133 = call <vilib>:"Add State(s) to Queue__jki_lib_state_machine.vi"("State(s) in (\"\")"=w313, "State(s) at Back (\"\")"=w307) -> ("States Out"=w312:string)  [unwired: 13 in]
            n134 = call <vilib>:"Add State(s) to Queue__jki_lib_state_machine.vi"("State(s) in Front (\"\")"=w312, "State(s) in (\"\")"=w319) -> ("States Out"=w318:string)  [unwired: 13 in]
          }
          frame "---------- Process ----------" {
            # "Template Separator\n(You can make a copy of, or modify, this frame)"
            n135 = call <vilib>:"Add State(s) to Queue__jki_lib_state_machine.vi"("State(s) in (\"\")"=w324) -> ("States Out"=w323:string)  [unwired: 14 in]
          }
          frame "Process: Sync" {
            n136 = Unbundle By Name(w332) -> ("Self Reference"=w328:refnum<class "Measurement.WavelengthSweeping.UI.lvclass">)
            n137 = call <vilib>:"WaitOnProcessSync.vi"("error in (no error)"=w327, "SMO"=w328) -> ("error out"=w326:errorcluster, "Don't run?"=w331:bool)  [unwired: 7 in, 1 out]
            n138 = Select(t="Data: Cleanup\nEvents: Unregister\nExit", s=w331, f="") -> (s? t:f=w325:string)
            n139 = call <vilib>:"Add State(s) to Queue__jki_lib_state_machine.vi"("State(s) in Front (\"\")"=w325, "State(s) in (\"\")"=w335) -> ("States Out"=w334:string)  [unwired: 13 in]
          }
          frame "---------- Events ----------" {
            # "Template Separator\n(You can make a copy of, or modify, this frame)"
            n140 = call <vilib>:"Add State(s) to Queue__jki_lib_state_machine.vi"("State(s) in (\"\")"=w340) -> ("States Out"=w339:string)  [unwired: 14 in]
          }
          frame "Events: Register" {
            # "Measurement base class Public Events"
            # "Base Class Protected Events"
            n141 = Unbundle By Name(w346) -> ("Self Reference"=w351:refnum<class "Measurement.WavelengthSweeping.UI.lvclass">)
            n142 = Unbundle By Name(w346) -> ("Dependencies.Measurement.WavelengthSweeping"=w345:refnum<class "Measurement.WavelengthSweeping.lvclass">)
            n143 = call <vilib>:"GetProtectedEvents.vi"("SMO"=w351) -> ("error out"=w347:errorcluster, "SMO Protected Events"=w352:T12)  [unwired: 8 in, 1 out]
            n144 = call "Measurement.GetPublicEventsRegistration.vi"("Measurement in"=w345) -> ("error out"=w341:errorcluster, "Measurement Public Events"=w342:refnum<event-registration>)  [unwired: 8 in, 1 out]
            n145 = register-events(w352) -> (reference out=w344:refnum<event-registration>, error out=w349:errorcluster)  [unwired: 2 in]
            n146 = Bundle("Event Registration Refnum"=w344, "Measurement Public Events"=w342) -> (w343:T13)  [unwired: 1 in]
            n147 = Merge Errors(w350, w349, w347, w341) -> (w348:errorcluster)
            n148 = call <vilib>:"Add State(s) to Queue__jki_lib_state_machine.vi"("State(s) in (\"\")"=w354) -> ("States Out"=w353:string)  [unwired: 14 in]
          }
          frame "Events: Unregister" {
            n149 = Unregister For Events(event registration refnum=w357, error in=w356) -> (error out=w355:errorcluster)
            n150 = call <vilib>:"Add State(s) to Queue__jki_lib_state_machine.vi"("State(s) in (\"\")"=w360) -> ("States Out"=w359:string)  [unwired: 14 in]
          }
          frame "---------- Action ----------" {
            n151 = Unbundle By Name(w363) -> ("Self Reference"=w361:refnum<class "Measurement.WavelengthSweeping.UI.lvclass">)
            n152 = Bundle By Name(cluster=w363, "Self Reference"=w361) -> (w362:T10)
            n153 = call <vilib>:"Add State(s) to Queue__jki_lib_state_machine.vi"("State(s) in (\"\")"=w367) -> ("States Out"=w366:string)  [unwired: 14 in]
          }
          frame "Action: Notify UI Closed" {
            # "Notify that the UI has been closed"
            n154 = Unbundle By Name(w370) -> ("Self Reference"=w371:refnum<class "Measurement.WavelengthSweeping.UI.lvclass">)
            n155 = call <vilib>:"Hide.vi"("error in (no error)"=w369, "SMO.UI"=w371) -> ("error out"=w368:errorcluster)  [unwired: 8 in, 1 out]
            n156 = call <vilib>:"Add State(s) to Queue__jki_lib_state_machine.vi"("State(s) in (\"\")"=w374) -> ("States Out"=w373:string)  [unwired: 14 in]
          }
        }
      }
    }
    frame Error {
    }
  }
  n157 = call-parent "Process.vi"("error in (no error)"=w8, "SMO.UI"=w7) -> ("error out"=w5:errorcluster, "SMO.UI out"=→"Measurement.WavelengthSweeping.UI out":refnum<class "Measurement.WavelengthSweeping.UI.lvclass">)  [unwired: 8 in]
  n158 = Merge Errors(w5, w4) -> (→"error out":errorcluster)
